vi "Initialize.vi"(8 "Error In":errorcluster, 10 "Output Directory Path":path, 11 "Source Directory Path":path) -> (0 "Error Out":errorcluster, 2 "All VIs":path[](array[path]), 3 "Doc Config":T1)   [LabVIEW 2011, in "LVH-Toolbox.lvlib" / "LVH-Documentation.lvlib"]
uses:
  LVH-Documentation.lvlib
  Private/Type Defs/Doc Config.ctl
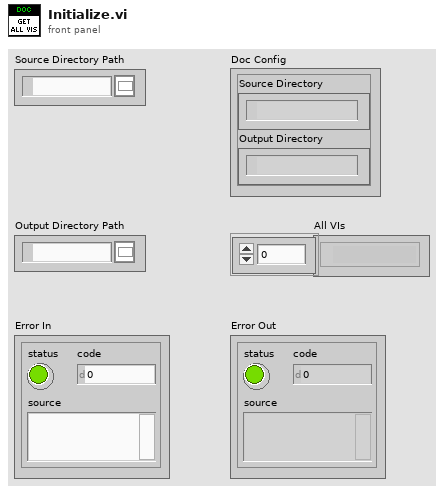
[diagram p1: front panel]
types:
  T1 = typedef "LVH-Toolbox.lvlib/LVH-Documentation.lvlib/Doc Config.ctl" = cluster{"Source Directory":path, "Output Directory":path}
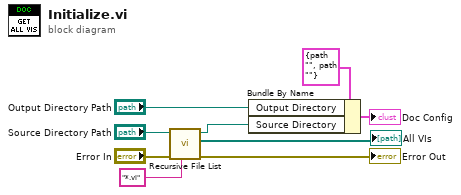
[diagram p0: block diagram]
diagram:
  n1 = call <vilib>:"Recursive File List.vi"("pattern"="*.vi", "error in (no error)"="Error In", "Folder Path"="Source Directory Path") -> ("error out"=→"Error Out":errorcluster, "All Files in Dir"=→"All VIs":path[], "dup Folder Path"=w3:path)  [unwired: 4 in, 2 out]
  n2 = Bundle By Name(cluster=T1 {"Source Directory"=path "", "Output Directory"=path ""} ("Doc Config"), "Output Directory"="Output Directory Path", "Source Directory"=w3) -> (→"Doc Config":T1)
